vi "reference_maker.vi"(8 "Raw_PPG":dbl[](array[numeric]), 11 "start_index":i32) -> (3 "reference":dbl[](array[numeric]))   [LabVIEW 2013]
panel:
  out "size":dbl
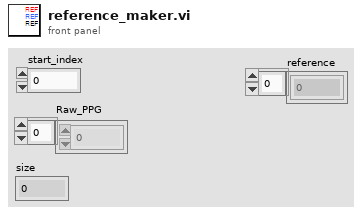
[diagram p1: front panel]
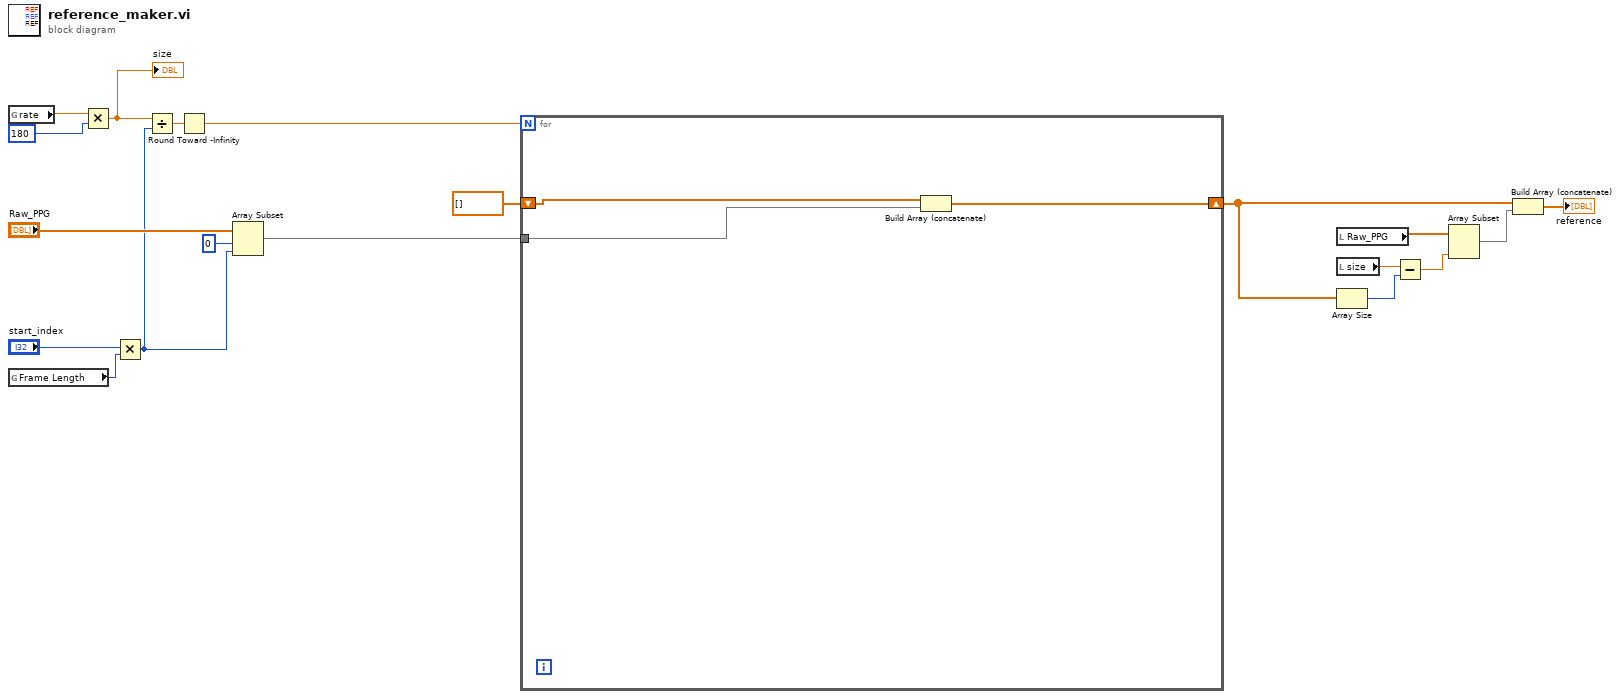
[diagram p0: block diagram]
diagram:
  n1 = global read "Control_Panel.vi" "rate"() -> (w15:dbl)
  n2 = global read "Control_Panel.vi" "Frame Length"() -> (w18:i32)
  n3 = Multiply(x=w15, y=180) -> (x*y=w8:dbl)
  "size" <- w8
  n4 = Multiply(x="start_index", y=w18) -> (x*y=w13:i32)
  n5 = Divide(x=w8, y=w13) -> (x/y=w12:dbl)
  n6 = Round Toward -Infinity(1:w12) -> (0:w9:dbl)
  n7 = Array Subset(array="Raw_PPG", index=0, length=w13) -> (w11:dbl[])
  n8 = for {
    N: w9 -> [_]
    tunnel: w11 -> [w22]
    shift-right: [w21] -> w3
    shift-left: dbl[] [] -> [w20]
    n9 = Build Array (concatenate)(w20, w22) -> (w21:dbl[])
  }
  n10 = local read "Raw_PPG"() -> (w4:dbl[])
  n11 = local read "size"() -> (w7:dbl)
  n12 = Array Size(array=w3) -> (size(s)=w6:i32)
  n13 = Subtract(x=w7, y=w6) -> (x-y=w5:dbl)
  n14 = Array Subset(array=w4, length=w5) -> (w2:dbl[])  [unwired: 1 in]
  n15 = Build Array (concatenate)(w3, w2) -> (→"reference":dbl[])
